vi "p04 comparacion 3 capas.vi"() -> ()   [LabVIEW 2013]
panel:
  in  "Vertical Pointer Slide 3":dbl(slide) scale=0.0..260.0
  in  "Vertical Pointer Slide 2":dbl(slide) scale=0.0..260.0
  in  "Vertical Pointer Slide":dbl(slide) scale=0.0..260.0
  out "Waveform Graph":dbl[][](graph)
  out "new picture 2":picture
  out "new picture":picture
  in  "path to JPEG file":path
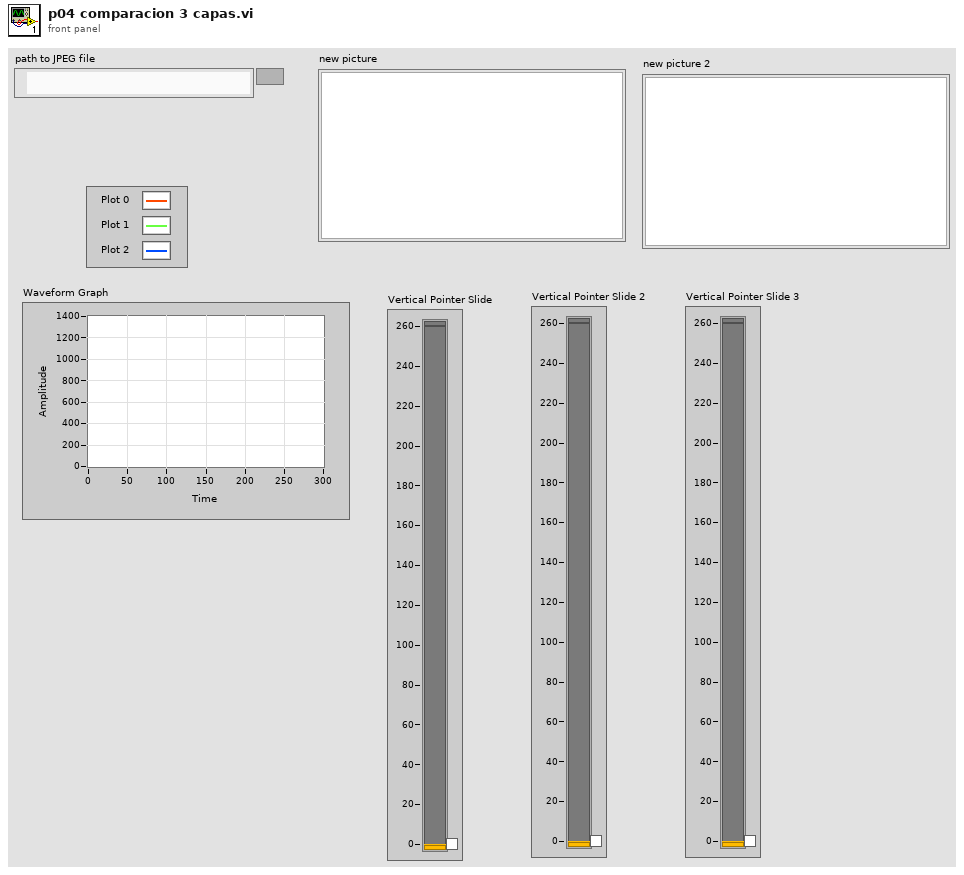
[diagram p1: front panel]
types:
  T1 = typedef "imagedata.ctl" = cluster{"image type":i32, "image depth":i32, "image":u8[], "mask":u8[], "colors":u32[], "Rectangle":cluster{"left":i16, "top":i16, "right":i16, "bottom":i16}}
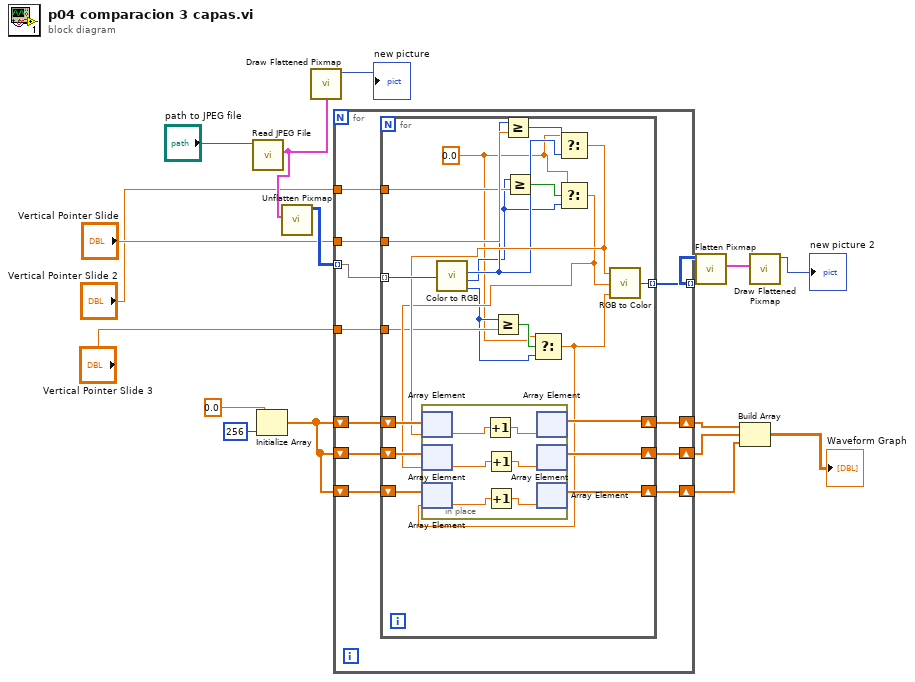
[diagram p0: block diagram]
diagram:
  n1 = call <vilib>:"Read JPEG File.vi"("path to JPEG file"="path to JPEG file") -> ("image data"=w15:T1)  [unwired: 8 in, 2 out]
  n2 = Initialize Array(0.0 ("element"), 256 ("dimension size")) -> (w8:dbl[])
  n3 = call <vilib>:"Unflatten Pixmap.vi"("image data"=w15) -> ("24-bit pixmap"=w14:u32[][])  [unwired: 4 in, 6 out]
  n4 = call <vilib>:"Draw Flattened Pixmap.vi"("image data"=w15) -> ("new picture"=→"new picture":picture)  [unwired: 8 in]
  n5 = for {
    tunnel: w14 -> [w28] mode=indexing
    tunnel: [w27] -> w13 mode=indexing
    shift-right: [w23] -> w7
    shift-left: w8 -> [w26]
    shift-right: [w22] -> w6
    shift-left: w8 -> [w25]
    shift-right: [w21] -> w5
    shift-left: w8 -> [w24]
    tunnel: "Vertical Pointer Slide" -> [w20]
    tunnel: "Vertical Pointer Slide 2" -> [w19]
    tunnel: "Vertical Pointer Slide 3" -> [w18]
    n6 = for {
      tunnel: w28 -> [w49] mode=indexing
      tunnel: [w48] -> w27 mode=indexing
      shift-right: [w44] -> w23
      shift-left: w26 -> [w47]
      shift-right: [w43] -> w22
      shift-left: w25 -> [w46]
      shift-right: [w42] -> w21
      shift-left: w24 -> [w45]
      tunnel: w20 -> [w40]
      tunnel: w19 -> [w38]
      tunnel: w18 -> [w35]
      w29 = 0.0 ("f")
      n7 = call <vilib>:"Color to RGB.vi"("Color"=w49) -> ("R"=w32:u8, "G"=w31:u8, "B"=w30:u8)  [unwired: 1 out]
      n8 = Greater Or Equal?(x=w30, y=w35) -> (x >= y?=w34:bool)
      n9 = Greater Or Equal?(x=w32, y=w40) -> (x >= y?=w41:bool)
      n10 = Greater Or Equal?(x=w31, y=w38) -> (x >= y?=w37:bool)
      n11 = Select(t=w29, s=w34, f=w30) -> (s? t:f=w33:dbl)
      n12 = Select(t=w29, s=w41, f=w32) -> (s? t:f=w39:dbl)
      n13 = Select(t=w29, s=w37, f=w31) -> (s? t:f=w36:dbl)
      n14 = in-place {
        n15 = in-place-array #1(w47, w39) -> (w55:dbl)
        n16 = in-place-array #2(w46, w36) -> (w53:dbl)
        n17 = in-place-array #3(w45, w33) -> (w51:dbl)
        n18 = Increment(x=w55) -> (x+1=w54:dbl)
        n19 = Increment(x=w53) -> (x+1=w52:dbl)
        n20 = Increment(x=w51) -> (x+1=w50:dbl)
        n21 = in-place-array #1(w54) -> (w44:dbl[])  [unwired: 1 out]
        n22 = in-place-array #2(w52) -> (w43:dbl[])  [unwired: 1 out]
        n23 = in-place-array #3(w50) -> (w42:dbl[])  [unwired: 1 out]
      }
      n24 = call <vilib>:"RGB to Color.vi"("B"=w33, "G"=w36, "R"=w39) -> ("Color"=w48:u32)
    }
  }
  n25 = call <vilib>:"Flatten Pixmap.vi"("24-bit pixmap"=w13) -> ("image data"=w12:T1)  [unwired: 10 in]
  n26 = Build Array(w7, w6, w5) -> (→"Waveform Graph":dbl[][])
  n27 = call <vilib>:"Draw Flattened Pixmap.vi"("image data"=w12) -> ("new picture"=→"new picture 2":picture)  [unwired: 8 in]
